vi "save_png.vi"(7 "shot name":string, 8 "error in (no error)":errorcluster, 9 "File Path":path, 10 "Image In":T1, 11 "ExperimentVariables in":refnum<class "ExperimentVariables.lvclass">) -> (0 "error out":errorcluster, 2 "Image Out (duplicate)":T1, 3 "ExperimentVariables out":refnum<class "ExperimentVariables.lvclass">)   [LabVIEW 2012]
uses:
  <vilib>/vision/Image Controls.llb/IMAQ Image.ctl
  ExperimentVariables/ExperimentVariables.lvclass
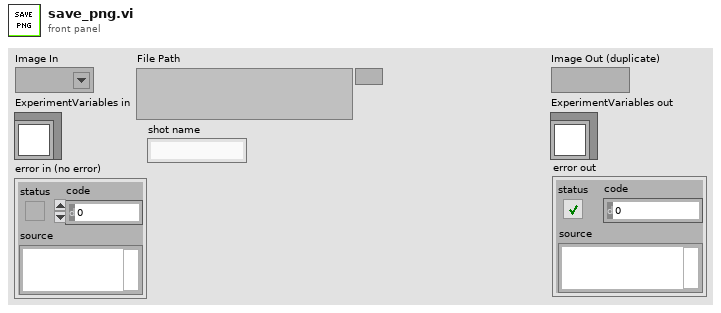
[diagram p1: front panel]
types:
  T1 = typedef "IMAQ Image.ctl" = refnum<image>
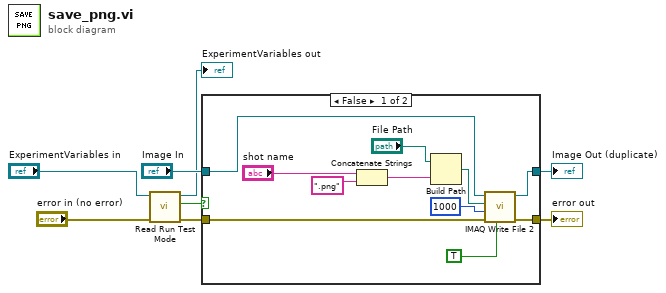
[diagram p0: block diagram]
diagram:
  n1 = call-dynamic "Read Run Test Mode.vi"("error in (no error)"="error in (no error)", "ExperimentVariables in"="ExperimentVariables in") -> ("error out"=w7:errorcluster, "Run Test Mode"=w8:bool, "ExperimentVariables out"=→"ExperimentVariables out":refnum<class "ExperimentVariables.lvclass">)  [unwired: 7 in]
  n2 = case shown="False" w8 {
    tunnel: w7 -> [w19 w20]
    tunnel: "Image In" -> [w18 w21]
    tunnel: [w17 w21] -> w6
    tunnel: [w16 w20] -> w1
    frame False {
      n3 = Concatenate Strings("shot name", ".png" ("string")) -> (w10:string)
      n4 = Build Path(base path="File Path", name or relative path=w10) -> (appended path=w12:path)
      n5 = call-poly "IMAQ Write File 2"("Use bit depth? (false)"=TRUE, "error in (no error)"=w19, "Image Quality"=u32 1000, "File Path"=w12, "Image"=w18) -> ("error out"=w16:errorcluster, "Image Out (duplicate)"=w17:T1)  [unwired: 5 in]
    }
    frame True {
    }
  }
  "Image Out (duplicate)" <- w6
  "error out" <- w1
